vi "Send command.vi"(8 "error in (no error)":errorcluster, 10 "Data":variant, 11 "command":string) -> (0 "error out":errorcluster)   [LabVIEW 2020, in "queue_display_loop_1.lvlib"]
uses:
  queue_display_loop_1.lvlib
  PTRL/dev_and_debug_tools/QueueMessage typedef.ctl
  PTRL/dev_and_debug_tools/dev_and_debug_tools.lvlib
panel:
  # "Development\ncontrols/indicators useful for development and testing, but which are not outputs of the VI"
  # "Input\nInputs to the VI"
  # "Output\nOutputs of the VI"
  # "Description\n\nBlank VI with error handling case. \n\nSummarize the use of this VI in this space."
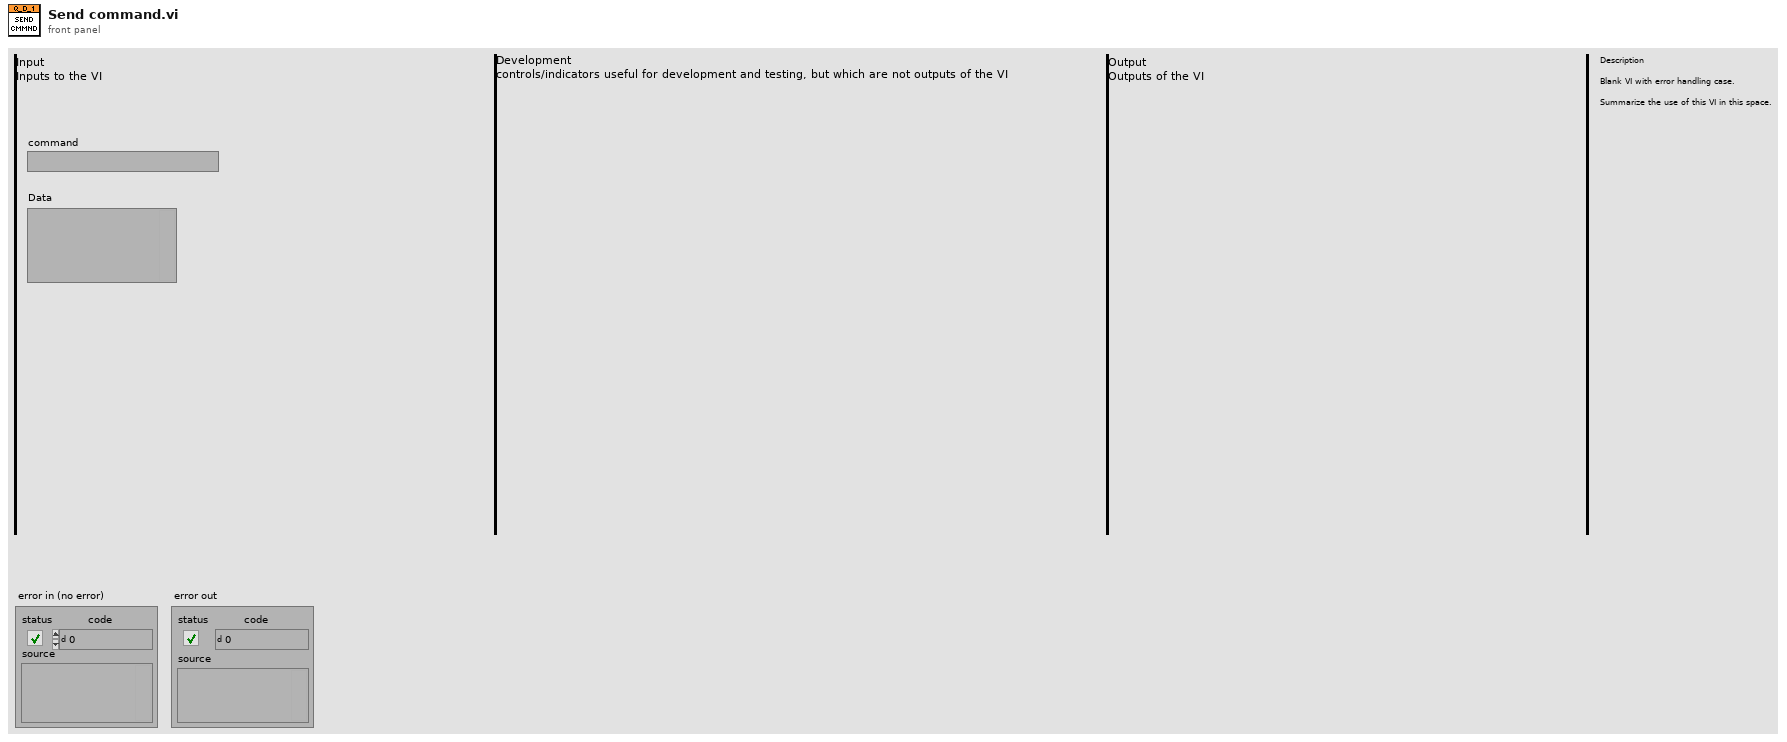
[diagram p1: front panel]
types:
  T1 = typedef "dev_and_debug_tools.lvlib/QueueMessage typedef.ctl" = cluster{"command":string, "data":variant}
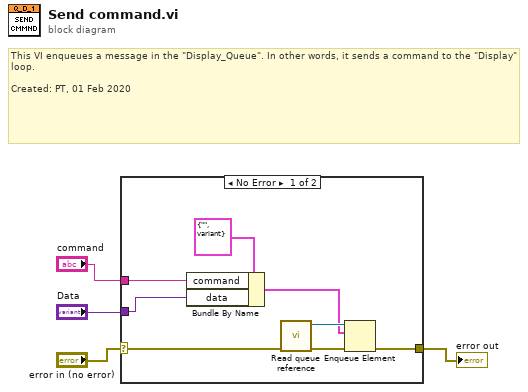
[diagram p0: block diagram]
diagram:
  # "This VI enqueues a message in the \"Display_Queue\". In other words, it sends a command to the \"Display\" loop.\n\nCreated: PT, 01 Feb 2020"
  n1 = case shown="No Error" "error in (no error)" {
    selector: "error in (no error)" -> [w12 w13]
    tunnel: [w11 w13] -> w3
    tunnel: "Data" -> [w6 _]
    tunnel: "command" -> [w5 _]
    frame No Error {
      n2 = Bundle By Name(cluster=T1 {"command"="", "data"=variant} ("element"), "command"=w5, "data"=w6) -> (w7:T1)
      n3 = call "Read queue reference.vi"("error in (no error)"=w12) -> ("error out"=w10:errorcluster, "ALA_Display_Queue ref"=w9:refnum<queue>)  [unwired: 9 in]
      n4 = Enqueue Element(queue=w9, element=w7, error in (no error)=w10) -> (error out=w11:errorcluster)  [unwired: 1 in, 2 out]
    }
    frame Error {
    }
  }
  "error out" <- w3
